vi "PM-GUI-Main.vi"(8 "error in":errorcluster, 11 "init_cluster":T1) -> (0 "error out":errorcluster, 3 "init_cluster out":T1)   [LabVIEW 2018]
uses:
  init-close/PM-init-data_cluster.ctl
  init-close/PM-init-user_events.ctl
  init-close/PM-common-heartrate_data.ctl
  init-close/PM-common-peak-detect_settings.ctl
  PM-GUI-loop_data.ctl
panel:
  in  "Peak Detection":bool
  in  "Bottom":dbl
  in  "Top":dbl
  in  "Acquire data?":bool
  in  "Stop":bool
  out "Last Update":timestamp
  in  "Reset collected wf":bool
  in  "Post Filtering remove":dbl
  in  "Collected signal size":u32
  in  "Reset avg":bool
  in  "Average over":u32
  out "heartrate avg":dbl
  out "Feedback":string
  in  "Tab Control":T3(tab)
  out "Filtered waveform":waveform(dbl)[](graph) caption="Filtered Signal"
  out "Raw signal":waveform(dbl)(graph)
  out "Live signal":waveform(dbl)(graph)
  out "heartrate":dbl
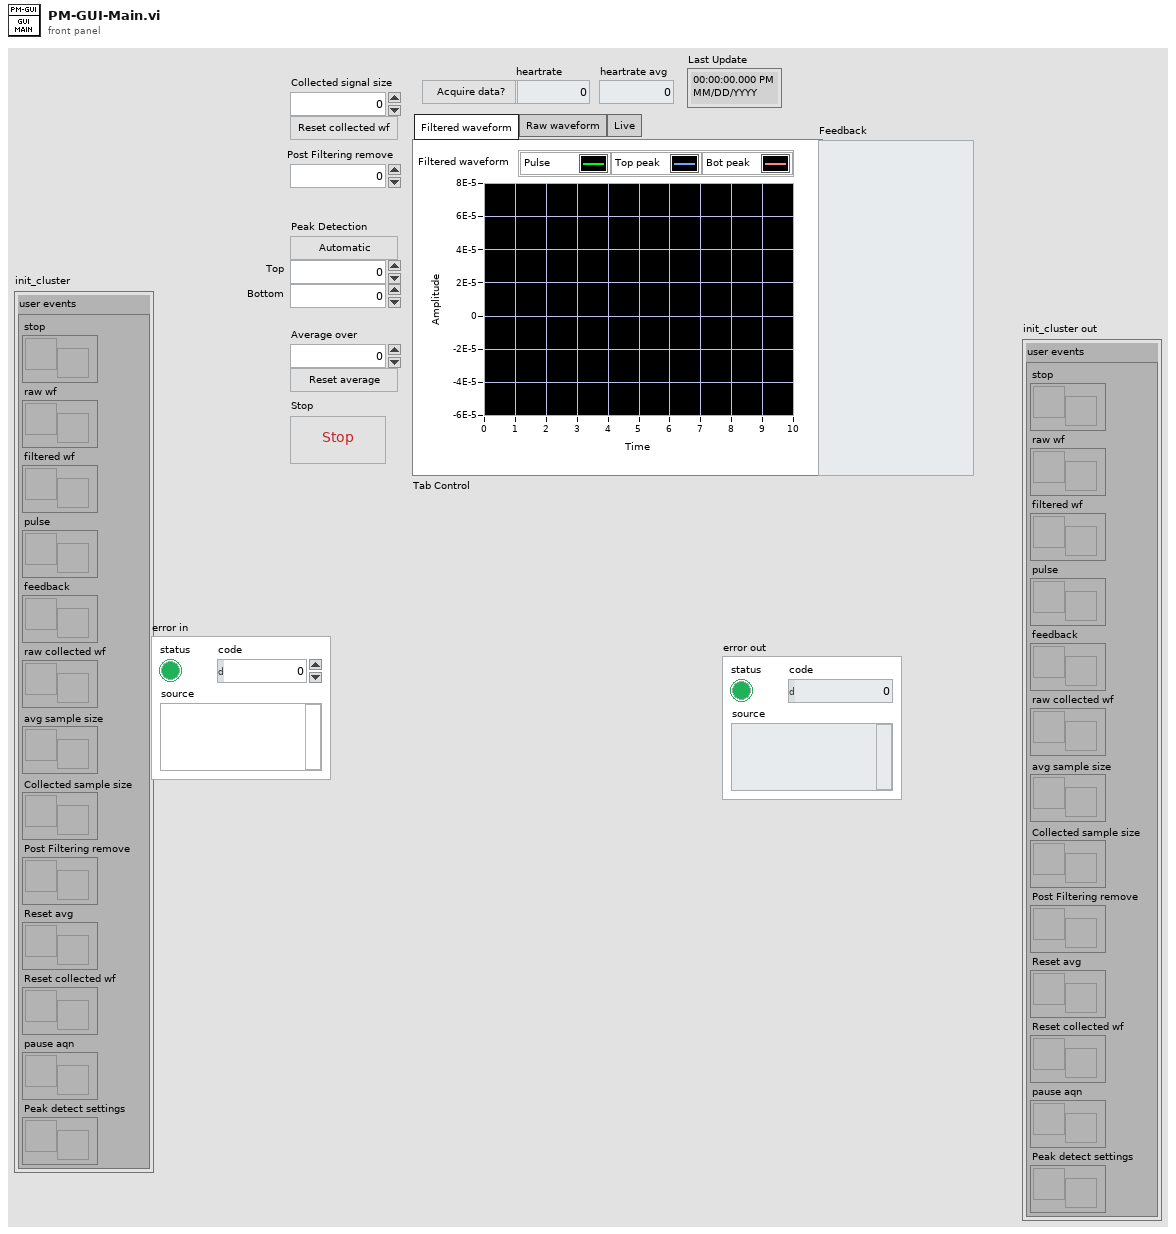
[diagram p1: front panel]
types:
  T1 = typedef "PM-init-data_cluster.ctl" = cluster{"user events":T2}
  T2 = typedef "PM-init-user_events.ctl" = cluster{"stop":refnum<user-event>, "raw wf":refnum<user-event>, "filtered wf":refnum<user-event>, "pulse":refnum<user-event>, "feedback":refnum<user-event>, "raw collected wf":refnum<user-event>, "avg sample size":refnum<user-event>, "Collected sample size":refnum<user-event>, "Post Filtering remove":refnum<user-event>, "Reset avg":refnum<user-event>, "Reset collected wf":refnum<user-event>, "pause aqn":refnum<user-event>, "Peak detect settings":refnum<user-event>}
  T3 = enum32{"Filtered waveform", "Raw waveform", "Live"}
  T4 = typedef "PM-GUI-loop_data.ctl" = cluster{"Stop event":refnum<user-event>, "avg sample size":refnum<user-event>, "Collected sample size":refnum<user-event>, "Post Filtering remove":refnum<user-event>, "Reset avg":refnum<user-event>, "Reset collected wf":refnum<user-event>, "pause aqn":refnum<user-event>, "Peak detect settings":refnum<user-event>}
  T5 = typedef "PM-common-peak-detect_settings.ctl" = cluster{"Top":dbl, "Bottom":dbl, "Peak Detection":bool}
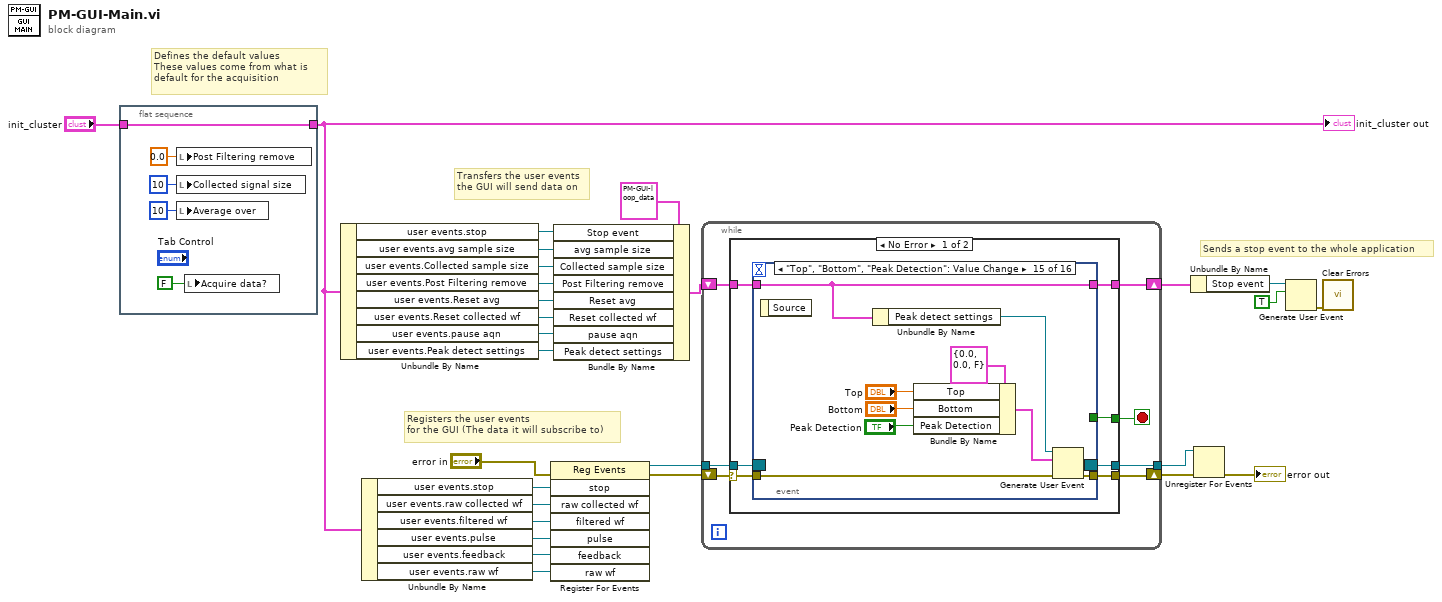
[diagram p0: block diagram]
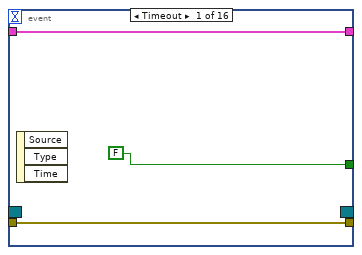
[diagram p2: hidden frame]
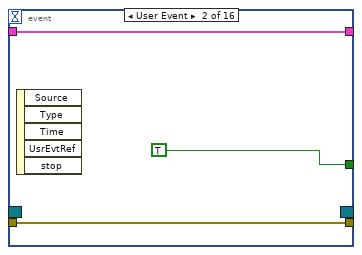
[diagram p3: hidden frame]
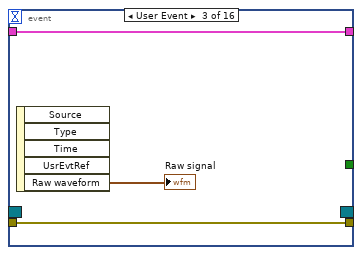
[diagram p4: hidden frame]
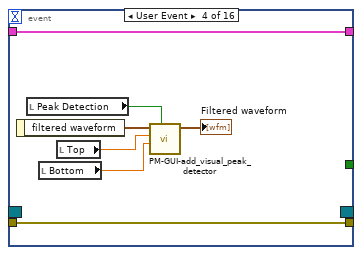
[diagram p5: hidden frame]
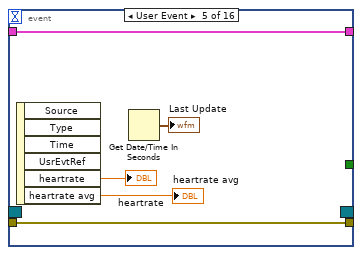
[diagram p6: hidden frame]
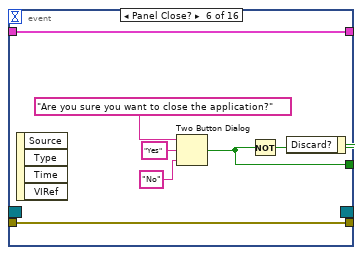
[diagram p7: hidden frame]
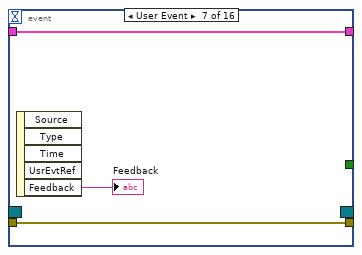
[diagram p8: hidden frame]
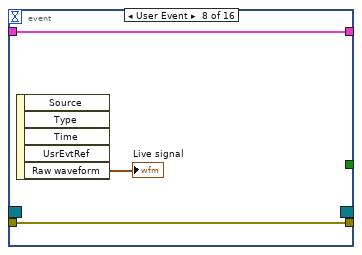
[diagram p9: hidden frame]
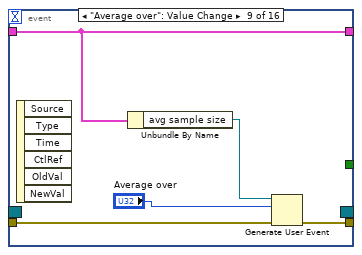
[diagram p10: hidden frame]
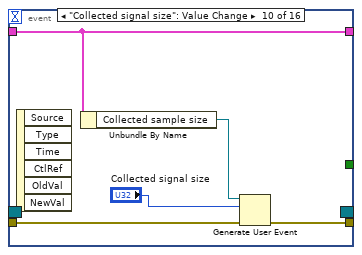
[diagram p11: hidden frame]
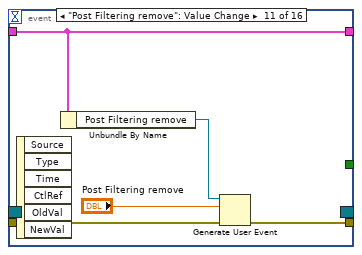
[diagram p12: hidden frame]
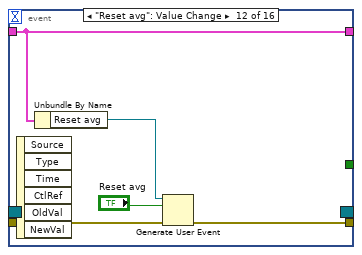
[diagram p13: hidden frame]
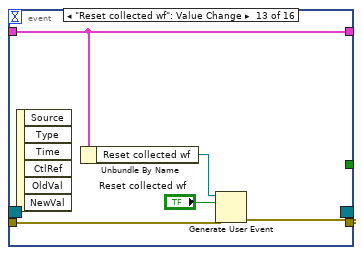
[diagram p14: hidden frame]
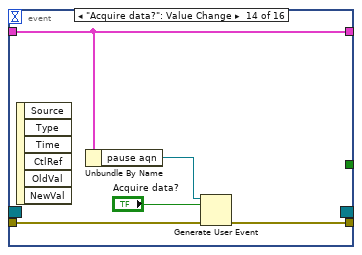
[diagram p15: hidden frame]
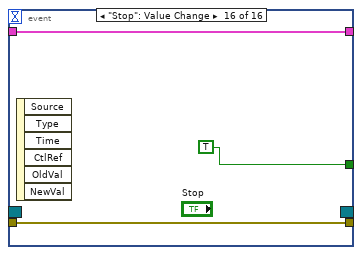
[diagram p16: hidden frame]
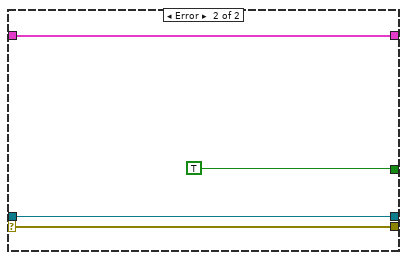
[diagram p17: hidden frame]
diagram:
  # "Sends a stop event to the whole application"
  # "Registers the user events\nfor the GUI (The data it will subscribe to)"
  # "Transfers the user events\nthe GUI will send data on"
  # "Defines the default values\nThese values come from what is \ndefault for the acquisition"
  n1 = flat-sequence {
    tunnel: "init_cluster" -> [w30]
    tunnel: [w30] -> w6
    frame #0 {
      n2 = local write "Post Filtering remove"(0.0 ("Post Filtering remove")) -> ()
      n3 = local write "Collected signal size"(u32 10 ("Collected signal size")) -> ()
      n4 = local write "Average over"(u32 10 ("Average over")) -> ()
      n5 = local write "Acquire data?"(FALSE ("pause aqn")) -> ()
    }
  }
  n6 = Unbundle By Name(w6) -> ("user events.stop"=w18:refnum<user-event>, "user events.avg sample size"=w12:refnum<user-event>, "user events.Collected sample size"=w11:refnum<user-event>, "user events.Post Filtering remove"=w10:refnum<user-event>, "user events.Reset avg"=w9:refnum<user-event>, "user events.Reset collected wf"=w8:refnum<user-event>, "user events.pause aqn"=w5:refnum<user-event>, "user events.Peak detect settings"=w1:refnum<user-event>)
  n7 = Unbundle By Name(w6) -> ("user events.stop"=w27:refnum<user-event>, "user events.raw collected wf"=w24:refnum<user-event>, "user events.filtered wf"=w23:refnum<user-event>, "user events.pulse"=w22:refnum<user-event>, "user events.feedback"=w21:refnum<user-event>, "user events.raw wf"=w13:refnum<user-event>)
  n8 = register-events(error in="error in", w27, w24, w23, w22, w21, w13) -> (reference out=w26:refnum<event-registration>, error out=w28:errorcluster)  [unwired: 1 in]
  n9 = Bundle By Name(cluster=T4 {"Stop event"=refnum, "avg sample size"=refnum, "Collected sample size"=refnum, "Post Filtering remove"=refnum, "Reset avg"=refnum, "Reset collected wf"=refnum, "pause aqn"=refnum, "Peak detect settings"=refnum} ("GUI-loop_data"), "Stop event"=w18, "avg sample size"=w12, "Collected sample size"=w11, "Post Filtering remove"=w10, "Reset avg"=w9, "Reset collected wf"=w8, "pause aqn"=w5, "Peak detect settings"=w1) -> (w19:T4)
  n10 = while {
    shift-right: [w38] -> w3
    shift-left: w28 -> [w40]
    tunnel: w26 -> [w37]
    shift-right: [w35] -> w17
    shift-left: w19 -> [w36]
    tunnel: [w34] -> w4
    stop <- w39 stop-if-true
    n11 = case shown="No Error" w40 {
      selector: w40 -> [w45 w126]
      tunnel: [w47 TRUE] -> w39
      tunnel: [w46 w126] -> w38
      tunnel: w37 -> [w44 w124]
      tunnel: w36 -> [w43 w125]
      tunnel: [w42 w125] -> w35
      tunnel: [w41 w124] -> w34
      frame No Error {
        n12 = event shown="[14] \"Top\", \"Bottom\", \"Peak Detection\": Value Change" {
          selector: w44 -> [_ _ _ _ _ _ _ _ _ _ _ _ _ _ _ _]
          dyn-events: [_ _ _ _ _ _ _ _ _ _ _ _ _ _ _ _] -> w41
          timeout: _ -> [_ _ _ _ _ _ _ _ _ _ _ _ _ _ _ _]
          tunnel: [FALSE TRUE _ _ _ w70 _ _ _ _ _ _ _ _ _ TRUE ("T button?")] -> w47
          tunnel: [w49 w53 w56 w63 w68 w75 w78 w81 w84 w89 w94 w99 w104 w109 w119 w123] -> w46
          tunnel: w45 -> [w49 w53 w56 w63 w68 w75 w78 w81 w85 w90 w95 w100 w105 w110 w120 w123]
          tunnel: w43 -> [w48 w51 w54 w62 w66 w69 w77 w80 w86 w91 w96 w101 w106 w111 w118 w122]
          tunnel: [w48 w51 w54 w62 w66 w69 w77 w80 w86 w91 w96 w101 w106 w111 w118 w122] -> w42
          event Timeout {
            n13 = event-data() -> ()  [unwired: 1 in, 3 out]
          }
          event User Event {
            n14 = event-data() -> ()  [unwired: 1 in, 5 out]
          }
          event User Event {
            n15 = event-data() -> ("Raw waveform"=→"Raw signal":waveform(dbl))  [unwired: 1 in, 4 out]
          }
          event User Event {
            n16 = event-data() -> ("filtered waveform"=w61:waveform(dbl))  [unwired: 1 in]
            n17 = local read "Peak Detection"() -> (w59:bool)
            n18 = local read "Bottom"() -> (w57:dbl)
            n19 = local read "Top"() -> (w58:dbl)
            n20 = call "PM-GUI-add_visual_peak_detector.vi"("Peak Detection"=w59, "Bottom"=w57, "Top"=w58, "waveform in"=w61) -> ("Waveforms out"=→"Filtered waveform":waveform(dbl)[])  [unwired: 7 in]
          }
          event User Event {
            n21 = event-data() -> ("heartrate"=→"heartrate":dbl, "heartrate avg"=→"heartrate avg":dbl)  [unwired: 1 in, 4 out]
            n22 = Get Date/Time In Seconds() -> (seconds since 1Jan1904=→"Last Update":timestamp)
          }
          event Panel Close? {
            n23 = event-data() -> ()  [unwired: 1 in, 4 out]
            n24 = Two Button Dialog(message="Are you sure you want to close the application?", 1:"No" ("F button name (\"Cancel\")"), 2:"Yes" ("T button name (\"OK\")")) -> (T button?=w70:bool)
            n25 = Not(x=w70) -> (.not. x?=w71:bool)
            n26 = event-data("Discard?"=w71) -> ()  [unwired: 1 in, 1 out]
          }
          event User Event {
            n27 = event-data() -> ("Feedback"=→"Feedback":string)  [unwired: 1 in, 4 out]
          }
          event User Event {
            n28 = event-data() -> ("Raw waveform"=→"Live signal":waveform(dbl))  [unwired: 1 in, 4 out]
          }
          event "Average over": Value Change {
            n29 = event-data() -> ()  [unwired: 1 in, 6 out]
            n30 = Unbundle By Name(w86) -> ("avg sample size"=w83:refnum<user-event>)
            n31 = Generate User Event(user event=w83, event data cluster="Average over", error in=w85) -> (error out=w84:errorcluster)  [unwired: 1 in, 1 out]
          }
          event "Collected signal size": Value Change {
            n32 = event-data() -> ()  [unwired: 1 in, 6 out]
            n33 = Unbundle By Name(w91) -> ("Collected sample size"=w88:refnum<user-event>)
            n34 = Generate User Event(user event=w88, event data cluster="Collected signal size", error in=w90) -> (error out=w89:errorcluster)  [unwired: 1 in, 1 out]
          }
          event "Post Filtering remove": Value Change {
            n35 = event-data() -> ()  [unwired: 1 in, 6 out]
            n36 = Unbundle By Name(w96) -> ("Post Filtering remove"=w93:refnum<user-event>)
            n37 = Generate User Event(user event=w93, event data cluster="Post Filtering remove", error in=w95) -> (error out=w94:errorcluster)  [unwired: 1 in, 1 out]
          }
          event "Reset avg": Value Change {
            n38 = event-data() -> ()  [unwired: 1 in, 6 out]
            n39 = Unbundle By Name(w101) -> ("Reset avg"=w98:refnum<user-event>)
            n40 = Generate User Event(user event=w98, event data cluster="Reset avg", error in=w100) -> (error out=w99:errorcluster)  [unwired: 1 in, 1 out]
          }
          event "Reset collected wf": Value Change {
            n41 = event-data() -> ()  [unwired: 1 in, 6 out]
            n42 = Unbundle By Name(w106) -> ("Reset collected wf"=w103:refnum<user-event>)
            n43 = Generate User Event(user event=w103, event data cluster="Reset collected wf", error in=w105) -> (error out=w104:errorcluster)  [unwired: 1 in, 1 out]
          }
          event "Acquire data?": Value Change {
            n44 = event-data() -> ()  [unwired: 1 in, 6 out]
            n45 = Unbundle By Name(w111) -> ("pause aqn"=w108:refnum<user-event>)
            n46 = Generate User Event(user event=w108, event data cluster="Acquire data?", error in=w110) -> (error out=w109:errorcluster)  [unwired: 1 in, 1 out]
          }
          event "Top", "Bottom", "Peak Detection": Value Change {
            n47 = event-data() -> ()  [unwired: 1 in, 1 out]
            n48 = Unbundle By Name(w118) -> ("Peak detect settings"=w117:refnum<user-event>)
            n49 = Bundle By Name(cluster=T5 {"Top"=0.0, "Bottom"=0.0, "Peak Detection"=FALSE} ("event data"), "Top"="Top", "Bottom"="Bottom", "Peak Detection"="Peak Detection") -> (w115:T5)
            n50 = Generate User Event(user event=w117, event data cluster=w115, error in=w120) -> (error out=w119:errorcluster)  [unwired: 1 in, 1 out]
          }
          event "Stop": Value Change {
            n51 = event-data() -> ()  [unwired: 1 in, 6 out]
          }
        }
      }
      frame Error {
      }
    }
  }
  n52 = Unbundle By Name(w17) -> ("Stop event"=w16:refnum<user-event>)
  n53 = Unregister For Events(event registration refnum=w4, error in=w3) -> (error out=→"error out":errorcluster)
  n54 = Generate User Event(user event=w16, event data cluster=TRUE ("event data")) -> (error out=w14:errorcluster)  [unwired: 2 in, 1 out]
  n55 = call <vilib>:"Clear Errors.vi"("error in (no error)"=w14) -> ()  [unwired: 5 in, 2 out]
  "init_cluster out" <- w6
